vi "testpsp.vi"() -> ()   [LabVIEW 2013, in "testvarlib.lvlib"]
uses:
  testvarlib.lvlib
  execution/Scan Engine runtime.lvclass
  <vilib>/NI/Tag Bus Module Framework/channel/channel classification.ctl
  configuration/url prefix.ctl
  <vilib>/NI/Tag Bus/tag/Data Type.ctl
  configuration/Scan Engine configuration.lvclass
  configuration/Scan Engine configuration.lvclass/Scan Engine configuration.ctl
  <vilib>/NI/Tag Bus/table/data polymorphs/write one/write Double.vi
  <vilib>/NI/Tag Bus/table/data polymorphs/read one/read Double.vi
  configuration/Write discover channels.vi
  configuration/Write configure scan engine.vi
  <vilib>/NI/Tag Bus/table/data table.lvlib
  <vilib>/NI/Tag Bus/tag/tag descriptor.lvclass
  <vilib>/NI/Tag Bus Module Framework/channel/TBM channel.lvclass
panel:
  in  "testvarin":dbl
  out "testvarout":dbl
  in  "testvaroutTB":dbl
  in  "stop":bool
  out "ok":bool
  out "testvarinTB":dbl
  out "final error":errorcluster
  out "output error":errorcluster
  out "input error":errorcluster
  out "init error":errorcluster
  out "correct execution settings":bool
  out "serialization problem":errorcluster
  out "invalid configuration":errorcluster
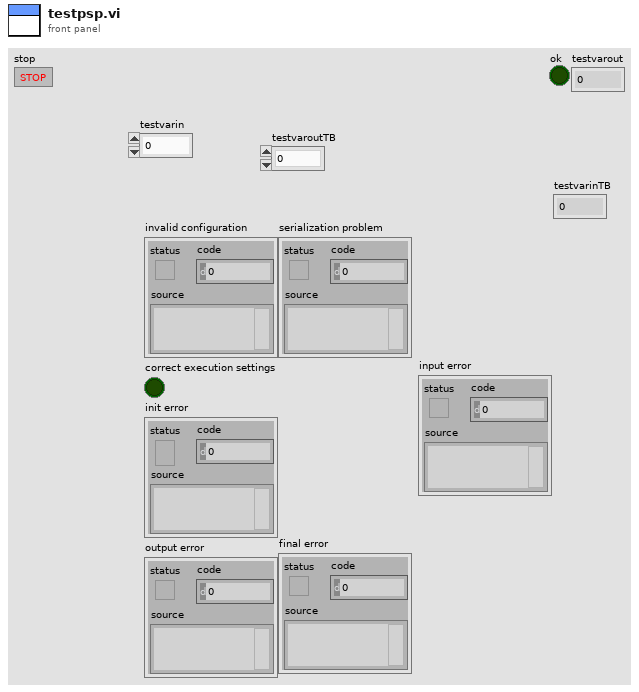
[diagram p1: front panel]
types:
  T1 = typedef "TBM channel.lvclass/channel classification.ctl" = enum16{"input data", "output data", "processing parameter", "processing result"}
  T2 = typedef "tag bus.lvlib/tag descriptor.lvclass/Data Type.ctl" = enum16{"Double", "Single", "I64", "I32", "I16", "I8", "U64", "U32", "U16", "U8", "Boolean", "String", "Array of Double", "Array of Single", "Array of I64", "Array of I32", "Array of I16", "Array of I8", "Array of U64", "Array of U32", "Array of U16", "Array of U8", "Array of Boolean", "Array of String"}
  T3 = typedef "Scan Engine configuration.lvclass/url prefix.ctl" = enum32{"ni.var.io://", "ni.var.psp://"}
  T4 = typedef "TBM channel.lvclass/data tables.ctl" = cluster{"input data":T5, "processing parameter":T5, "processing result":T5, "output data":T5}
  T5 = typedef "tag bus.lvlib/dictionary table pair.ctl" = cluster{"data dictionary":refnum<class "data dictionary.lvclass">, "data table":T6}
  T6 = typedef "tag bus.lvlib/data table.lvlib/data table.ctl" = cluster{"Double":dbl[], "Single":sgl[], "I64":i64[], "I32":i32[], "I16":i16[], "I8":i8[], "U64":u64[], "U32":u32[], "U16":u16[], "U8":u8[], "Boolean":bool[], "String":string[], "Array of Double":cluster{"DBL Array":dbl[]}[], "Array of Single":cluster{"SGL Array":sgl[]}[], "Array of I64":cluster{"I64 Array":i64[]}[], "Array of I32":cluster{"I32 Array":i32[]}[], "Array of I16":cluster{"I16 Array":i16[]}[], "Array of I8":cluster{"I8 Array":i8[]}[], "Array of U64":cluster{"U64 Array":u64[]}[], "Array of U32":cluster{"U32 Array":u32[]}[], "Array of U16":cluster{"U16 Array":u16[]}[], "Array of U8":cluster{"U8 Array":u8[]}[], "Array of Boolean":cluster{"Boolean Array":bool[]}[], "Array of String":cluster{"String Array":string[]}[]}
  T7 = typedef "TBM module execution interface.lvclass/execution settings.ctl" = cluster{"reads inputs":bool, "processes data":bool, "writes outputs":bool}
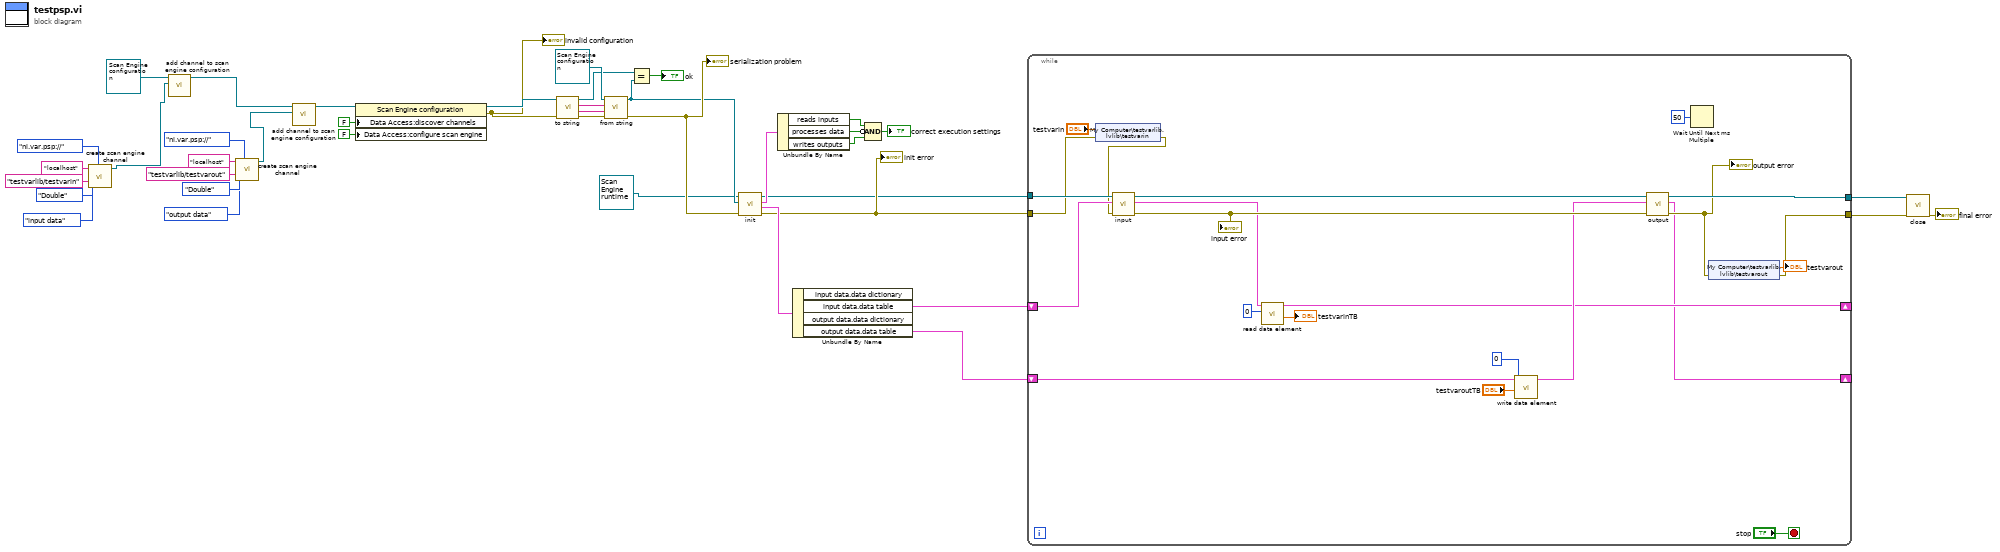
[diagram p0: block diagram]
diagram:
  n1 = call "create scan engine channel.vi"("URL"=url_prefix."ni.var.psp://", "channel classification"=channel_classification."input data", "data type"=Data_Type."Double", "variable name"="testvarlib/testvarin", "hostname"="localhost") -> ("channel"=w8:refnum<class "TBM channel.lvclass">)  [unwired: 6 in]
  n2 = call "add channel to scan engine configuration.vi"("channel"=w8, "Scan Engine configuration in"=refnum<class "Scan Engine configuration.lvclass"> refnum ("Scan Engine configuration")) -> ("Scan Engine configuration out"=w19:refnum<class "Scan Engine configuration.lvclass">)  [unwired: 8 in, 1 out]
  n3 = call "create scan engine channel.vi"("URL"=url_prefix."ni.var.psp://", "channel classification"=channel_classification."output data", "data type"=Data_Type."Double", "variable name"="testvarlib/testvarout", "hostname"="localhost") -> ("channel"=w7:refnum<class "TBM channel.lvclass">)  [unwired: 6 in]
  n4 = call "add channel to scan engine configuration.vi"("channel"=w7, "Scan Engine configuration in"=w19) -> ("Scan Engine configuration out"=w20:refnum<class "Scan Engine configuration.lvclass">)  [unwired: 8 in, 1 out]
  n5 = property class="Scan Engine configuration"(reference=w20, "Data Access:discover channels"=FALSE ("discover channels"), "Data Access:configure scan engine"=FALSE ("configure scan engine")) -> (reference out=w24:refnum<class "Scan Engine configuration.lvclass">, error out=w23:errorcluster)  [unwired: 1 in]
  "invalid configuration" <- w23
  n6 = call-dynamic "to string.vi"("error in"=w23, "Scan Engine configuration in"=w24) -> ("error out"=w39:errorcluster, "data"=w40:string, "version"=w41:string, "Scan Engine configuration out"=w4:refnum<class "Scan Engine configuration.lvclass">)  [unwired: 6 in]
  n7 = call-dynamic "from string.vi"("error in"=w39, "data"=w40, "version"=w41, "Scan Engine configuration in"=refnum<class "Scan Engine configuration.lvclass"> refnum ("Scan Engine configuration")) -> ("error out"=w38:errorcluster, "Scan Engine configuration out"=w3:refnum<class "Scan Engine configuration.lvclass">)  [unwired: 6 in]
  "serialization problem" <- w38
  n8 = Equal?(x=w4, y=w3) -> (x = y?=→"ok":bool)
  n9 = call-dynamic "init.vi"("error in"=w38, "TBM module configuration in"=w3, "Scan Engine runtime in"=refnum<class "Scan Engine runtime.lvclass"> refnum ("Scan Engine runtime")) -> ("error out"=w31:errorcluster, "data allocations"=w32:T4, "execution settings"=w37:T7, "Scan Engine runtime out"=w29:refnum<class "Scan Engine runtime.lvclass">)  [unwired: 5 in]
  "init error" <- w31
  n10 = Unbundle By Name(w37) -> ("reads inputs"=w34:bool, "processes data"=w36:bool, "writes outputs"=w35:bool)
  n11 = Unbundle By Name(w32) -> ("input data.data table"=w30:T6, "output data.data table"=w28:T6)  [unwired: 2 out]
  n12 = Compound Arithmetic op=AND(w34, invert w36, w35) -> (→"correct execution settings":bool)
  n13 = while {
    tunnel: w31 -> [w49]
    tunnel: w29 -> [w62]
    tunnel: [w57] -> w27
    tunnel: [w46] -> w26
    shift-right: [w43] -> _
    shift-left: w30 -> [w63]
    shift-right: [w42] -> _
    shift-left: w28 -> [w61]
    stop <- "stop" stop-if-true
    n14 = shared-variable "My Computer\\testvarlib.lvlib\\testvarin"("testvarin", error in=w49) -> (error out=w48:errorcluster)
    n15 = call-dynamic "input.vi"("error in"=w48, "data table in"=w63, "Scan Engine runtime in"=w62) -> ("error out"=w60:errorcluster, "data table out"=w56:T6, "Scan Engine runtime out"=w59:refnum<class "Scan Engine runtime.lvclass">)  [unwired: 6 in]
    "input error" <- w60
    n16 = call-poly <vilib>:"read data element.vi"("index"=0, "data table in"=w56) -> ("value"=→"testvarinTB":dbl, "data table out"=w43:T6)  [unwired: 8 in]
    n17 = call-poly <vilib>:"write data element.vi"("value"="testvaroutTB", "index"=0, "data table in"=w61) -> ("data table out"=w58:T6)  [unwired: 8 in]
    n18 = call-dynamic "output.vi"("error in"=w60, "data table in"=w58, "Scan Engine runtime in"=w59) -> ("error out"=w47:errorcluster, "data table out"=w42:T6, "Scan Engine runtime out"=w57:refnum<class "Scan Engine runtime.lvclass">)  [unwired: 6 in]
    "output error" <- w47
    n19 = Wait Until Next ms Multiple(millisecond multiple=u32 50) -> ()  [unwired: 1 out]
    n20 = shared-variable "My Computer\\testvarlib.lvlib\\testvarout"(error in=w47) -> (→"testvarout":dbl, error out=w46:errorcluster)
  }
  n21 = call-dynamic "close.vi"("error in"=w26, "Scan Engine runtime in"=w27) -> ("error out"=→"final error":errorcluster)  [unwired: 9 in]
